vi "Host-UART-State-Machine-Tester.vi"() -> ()   [LabVIEW 2017]
uses:
  UART.States.ctl
  <vilib>/FPGAPlugInAG/Dynamic/niLvFpga_Download_Dynamic.vi
  <vilib>/Utility/error.llb/Error Cluster From Error Code.vi
  <vilib>/rvi/errors/niLvFpgaAdjustHostInterfaceError.vi
  <vilib>/FPGAPlugInAG/Dynamic/niLvFpga_Run_Dynamic.vi
  <vilib>/FPGAPlugInAG/Dynamic/niLvFpga_Close_Dynamic.vi
  <vilib>/rvi/interface/nirviMethod/nirviMethod.xnode
  <vilib>/rvi/interface/nirviReadWriteControl/nirviReadWriteControl.xnode
  <vilib>/rvi/interface/nirviCloseFPGA/nirviCloseFPGA.xnode
  <vilib>/FPGAPlugInAG/Dynamic/niLvFpga_ReadFifo_Dynamic.vi
  <vilib>/rvi/errors/niLvFpgaMergeErrorWithErrorCode.vi
  NiFpgaLv.dll
  <vilib>/rvi/interface/Simulation/niFpgaSimulationCallBeginRW.vi
  <vilib>/FPGAPlugInAG/Dynamic/niLvFpga_WriteFifo_Dynamic.vi
panel:
  out "FPGA\nReady":bool
  in  "Download\nBitfile?":bool=TRUE
  in  "Data to Send":string="A"
  in  "Receive":bool
  in  "Transmit":bool
  in  "Bitfile path":path=path "Z:/work/git/LabVIEW_Fpga/06_MicroBlaze/05_UART/ProjectExportForVivado/FpgaUart/FpgaUart.lvbitx"
  out "Data Received":string
  out "error out":errorcluster
  in  "stop":bool
  in  "error in":errorcluster
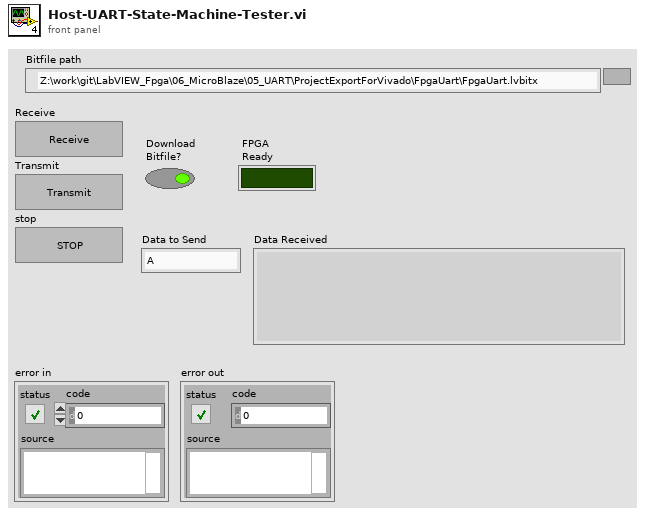
[diagram p1: front panel]
types:
  T1 = typedef "UART.States.ctl" = enum16{"Open-Fpga", "Poll-RX", "Transmit", "Close-Fpga"}
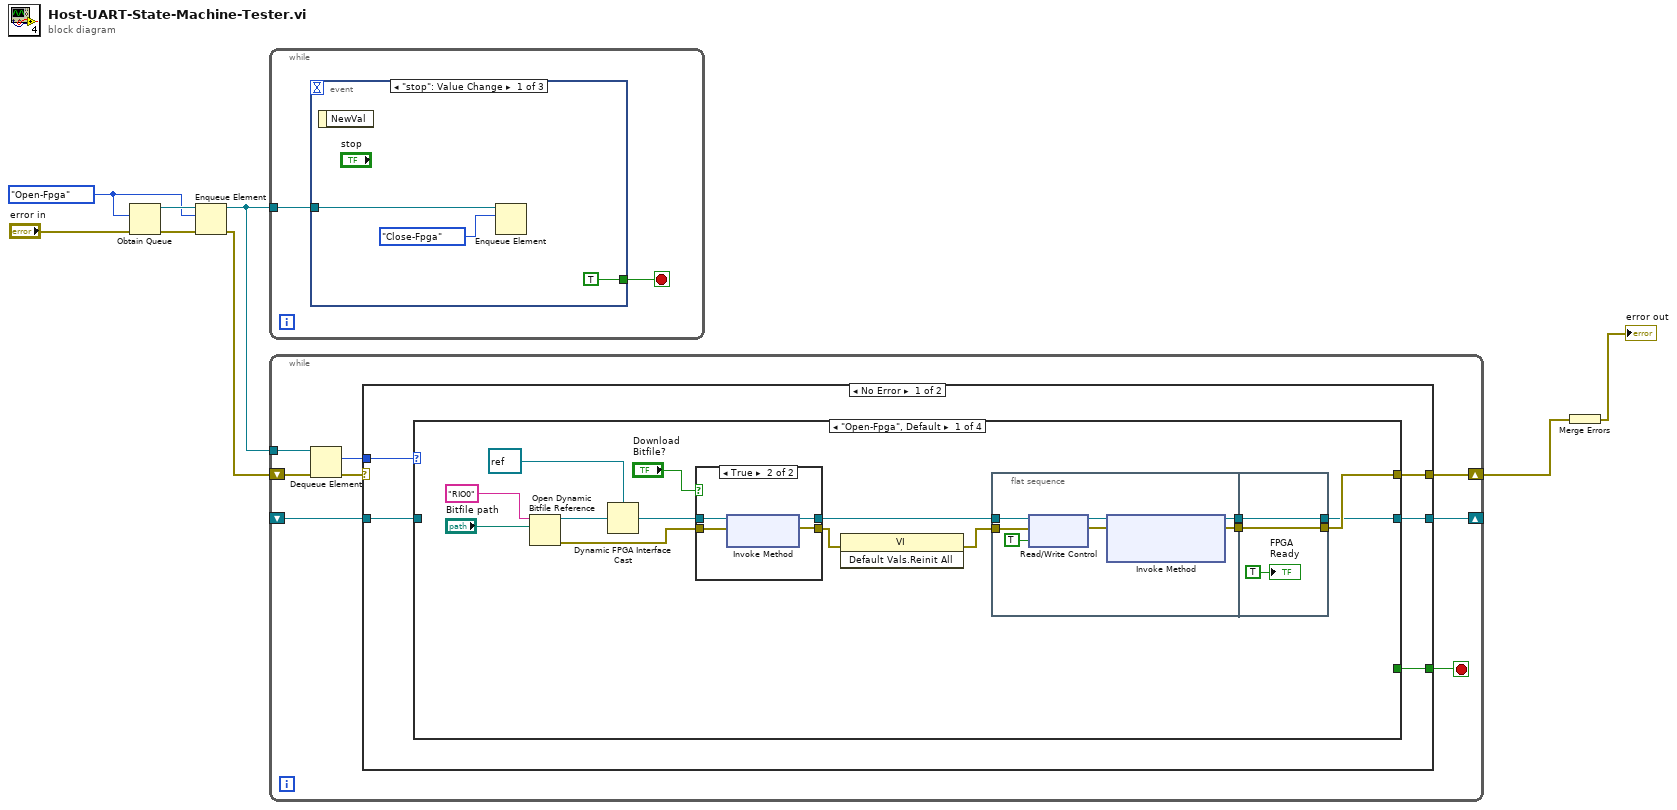
[diagram p0: block diagram]
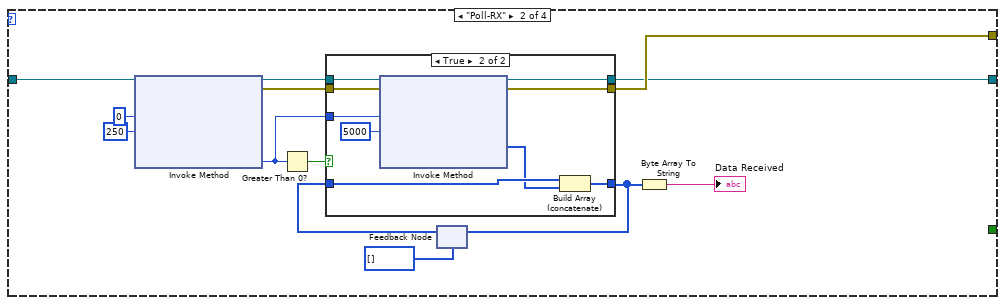
[diagram p3: hidden frame]
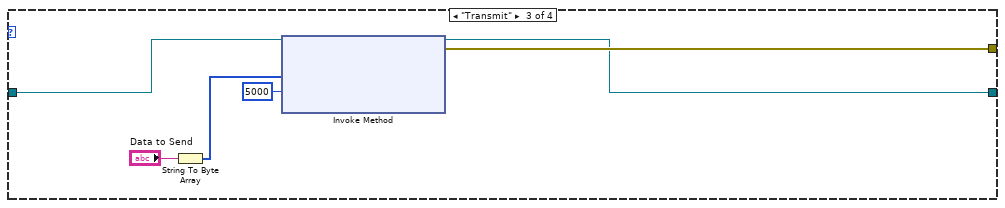
[diagram p5: hidden frame]
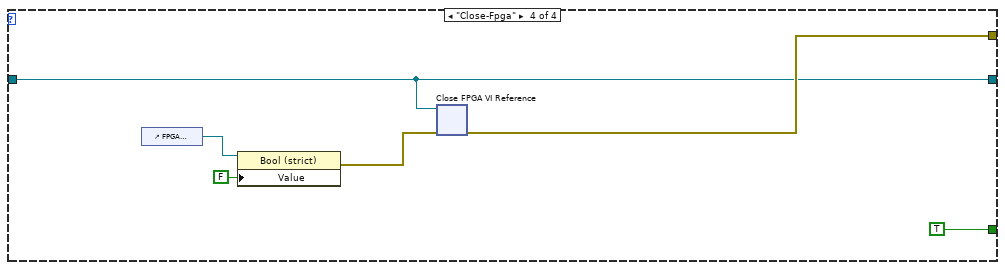
[diagram p6: hidden frame]
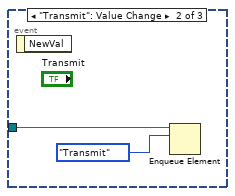
[diagram p8: hidden frame]
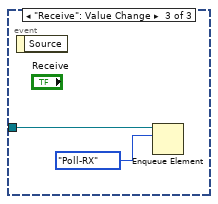
[diagram p9: hidden frame]
diagram:
  w5 = UART.States."Open-Fpga"
  n1 = Obtain Queue(element data type=w5, error in (no error)="error in") -> (queue out=w7:refnum<queue>, error out=w6:errorcluster)  [unwired: 3 in, 1 out]
  n2 = Enqueue Element(queue=w7, element=w5, error in (no error)=w6) -> (queue out=w4:refnum<queue>, error out=w3:errorcluster)  [unwired: 1 in, 1 out]
  n3 = while {
    tunnel: w4 -> [w10]
    stop <- w9 stop-if-true
    n4 = event shown="[0] \"stop\": Value Change" {
      selector: _ -> [_ _ _]
      dyn-events: _ -> [_ _ _]
      timeout: _ -> [_ _ _]
      tunnel: w10 -> [w13 w14 w16]
      tunnel: [TRUE _ _] -> w9
      event "stop": Value Change {
        n5 = event-data() -> ()  [unwired: 1 in, 1 out]
        n6 = Enqueue Element(queue=w13, element=UART.States."Close-Fpga") -> ()  [unwired: 2 in, 3 out]
      }
      event "Transmit": Value Change {
        n7 = event-data() -> ()  [unwired: 1 in, 1 out]
        n8 = Enqueue Element(queue=w14, element=UART.States."Transmit") -> ()  [unwired: 2 in, 3 out]
      }
      event "Receive": Value Change {
        n9 = event-data() -> ()  [unwired: 1 in, 1 out]
        n10 = Enqueue Element(queue=w16, element=UART.States."Poll-RX") -> ()  [unwired: 2 in, 3 out]
      }
    }
  }
  n11 = while {
    tunnel: w4 -> [w23]
    shift-right: [w20] -> w2
    shift-left: w3 -> [w22]
    shift-right: [w19] -> _
    shift-left: _ -> [w18]
    stop <- w21 stop-if-true
    n12 = Dequeue Element(queue=w23, error in (no error)=w22) -> (element=w24:T1, error out=w25:errorcluster)  [unwired: 1 in, 2 out]
    n13 = case shown="No Error" w25 {
      selector: w25 -> [_ w99]
      tunnel: w24 -> [w30 _]
      tunnel: [w29 _] -> w21
      tunnel: [w28 w99] -> w20
      tunnel: w18 -> [w27 w98]
      tunnel: [w26 w98] -> w19
      frame No Error {
        n14 = case shown="\"Open-Fpga\", Default" w30 {
          tunnel: [_ _ _ TRUE] -> w29
          tunnel: [w44 w67 w90 w96] -> w28
          tunnel: w27 -> [_ w61 w86 w95]
          tunnel: [w42 w62 w87 w95] -> w26
          frame "Open-Fpga", Default {
            n15 = Open Dynamic Bitfile Reference(0:"RIO0" ("Device address"), 1:"Bitfile path") -> (5:w35:refnum<k20>, 8:w33:errorcluster)  [unwired: 3 in]
            n16 = Dynamic FPGA Interface Cast(Session In=refnum<k20> refnum ("FPGA Interface"), Type=w35) -> (Session Out=w34:refnum<k20>)
            n17 = case shown="True" "Download\nBitfile?" {
              tunnel: w34 -> [w55 w60]
              tunnel: [w55 w59] -> w43
              tunnel: w33 -> [w56 w58]
              tunnel: [w56 w57] -> w38
              frame False {
              }
              frame True {
                n18 = xnode "Invoke Method"("FPGA VI Reference In"=w60, "error in"=w58) -> ("FPGA VI Reference Out"=w59:refnum<k20>, "error out"=w57:errorcluster)
              }
            }
            n19 = invoke class="VI" method="Default Vals.Reinit All"(error in=w38) -> (error out=w37:errorcluster)  [unwired: 2 in, 2 out]
            n20 = flat-sequence {
              tunnel: [w48] -> w40
              tunnel: [w46] -> w39
              tunnel: w43 -> [w47]
              tunnel: w37 -> [w45]
              tunnel: [w53] -> w42
              tunnel: [w54] -> w44
              tunnel: w40 -> [w54]
              tunnel: w39 -> [w53]
              frame #0 {
                n21 = xnode "Read/Write Control"("FPGA VI Reference In"=w47, "error in"=w45, "reset_rtl"=TRUE) -> ("FPGA VI Reference Out"=w51:refnum<k20>, "error out"=w49:errorcluster)
                n22 = xnode "Invoke Method"("FPGA VI Reference In"=w51, "error in"=w49) -> ("FPGA VI Reference Out"=w46:refnum<k20>, "error out"=w48:errorcluster)  [unwired: 1 in]
              }
              frame #1 {
                "FPGA\nReady" <- TRUE ("FPGA\nReady")
              }
            }
          }
          frame "Poll-RX" {
            n23 = xnode "Invoke Method"("FPGA VI Reference In"=w61, "Number of Elements"=u32 0, "Timeout (ms)"=250) -> ("FPGA VI Reference Out"=w70:refnum<k20>, "error out"=w69:errorcluster, "Elements Remaining"=w68:u32)  [unwired: 1 in, 1 out]
            n24 = Greater Than 0?(x=w68) -> (x > 0?=w71:bool)
            n25 = feedback #1(u8[] []) -> (w66:u8[])
            n26 = case shown="True" w71 {
              tunnel: w70 -> [w74 w85]
              tunnel: w69 -> [w75 w84]
              tunnel: w68 -> [_ w83]
              tunnel: w66 -> [w76 w81]
              tunnel: [w76 w79] -> w64
              tunnel: [w74 w78] -> w62
              tunnel: [w75 w77] -> w67
              frame False {
              }
              frame True {
                n27 = xnode "Invoke Method"("FPGA VI Reference In"=w85, "error in"=w84, "Number of Elements"=w83, "Timeout (ms)"=5000) -> ("FPGA VI Reference Out"=w78:refnum<k20>, "error out"=w77:errorcluster, "Data"=w80:u8[])  [unwired: 1 out]
                n28 = Build Array (concatenate)(w81, w80) -> (w79:u8[])
              }
            }
            n29 = feedback-in #1(w64) -> ()
            n30 = Byte Array To String(unsigned byte array=w64) -> (string=→"Data Received":string)
          }
          frame "Transmit" {
            n31 = String To Byte Array(string="Data to Send") -> (unsigned byte array=w89:u8[])
            n32 = xnode "Invoke Method"("FPGA VI Reference In"=w86, "Data"=w89, "Timeout (ms)"=5000) -> ("FPGA VI Reference Out"=w87:refnum<k20>, "error out"=w90:errorcluster)  [unwired: 1 in, 1 out]
          }
          frame "Close-Fpga" {
            n33 = control-ref of="FPGA\nReady"() -> (w94:refnum<vi>)
            n34 = property class="Bool (strict)"(reference=w94, "Value"=FALSE) -> (error out=w92:errorcluster)  [unwired: 1 in, 1 out]
            n35 = xnode "Close FPGA VI Reference"("FPGA VI Reference In"=w95, "error in"=w92) -> ("error out"=w96:errorcluster)
          }
        }
      }
      frame Error {
      }
    }
  }
  n36 = Merge Errors(w2) -> (→"error out":errorcluster)
